vi "FillSurfaceRect.vi"(7 "Entire Surface (F)":bool, 8 "No Error":errorcluster, 9 "color":u32, 10 "rect":T1, 11 "dst [SDL_Surface *]":i64) -> (0 "error out":errorcluster)   [LabVIEW 2024, in "SDL3.lvlib" / "Surface.lvlib"]
doc: "<B>Summary</B>\nPerform a fast fill of a rectangle with a specific color.\n\n<B>Remarks</B>\ncolor should be a pixel of the format used by the surface, and can be generated by SDL_MapRGB() or SDL_MapRGBA(). If the color value contains an alpha component then the destination is simply filled with that alpha information, no blending takes place.\n\nIf there is a clip rectangle set on the destination (set via SDL_SetSurfaceClipRect()), then this function will fill based on the intersection of the clip rectangle and rect."
uses:
  Surface.lvlib
  Rect/Rect--cluster.ctl
  Error/Error.lvlib
  Lib/SDL3-32.dll
  Rect/Rect.lvlib
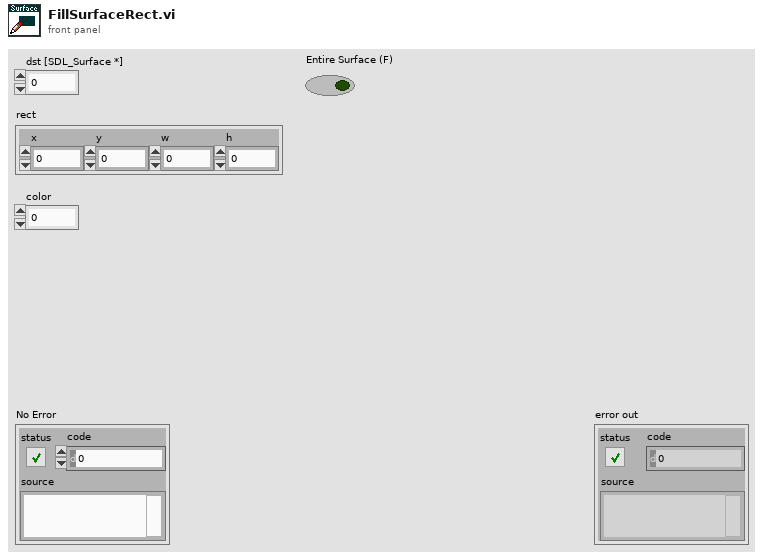
[diagram p1: front panel]
types:
  T1 = typedef "SDL3.lvlib/Rect.lvlib/Rect--cluster.ctl" = cluster{"x":i32, "y":i32, "w":i32, "h":i32}
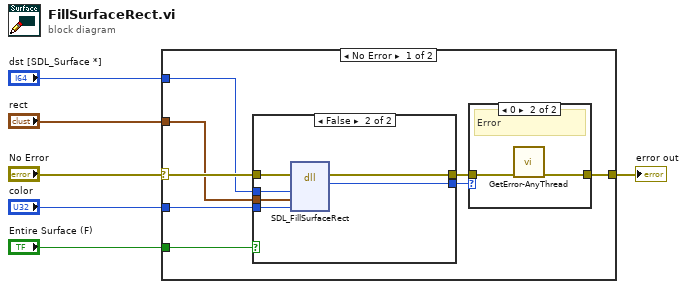
[diagram p0: block diagram]
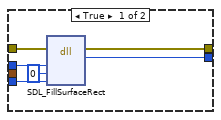
[diagram p2: hidden frame]
diagram:
  n1 = case shown="No Error" "No Error" {
    selector: "No Error" -> [w14 w30]
    tunnel: [w12 w30] -> w5
    tunnel: "dst [SDL_Surface *]" -> [w10 _]
    tunnel: "rect" -> [w9 _]
    tunnel: "color" -> [w8 _]
    tunnel: "Entire Surface (F)" -> [w7 _]
    frame No Error {
      n2 = case shown="False" w7 {
        tunnel: w14 -> [w20 w26]
        tunnel: [w19 w25] -> w13
        tunnel: [w18 w24] -> w11
        tunnel: w10 -> [w17 w23]
        tunnel: w9 -> [_ w22]
        tunnel: w8 -> [w16 w21]
        frame True {
          n3 = dll-call lib="C:/Users/Thomas/Documents/Projects/LV-SDL3/Lib/SDL3-*.*" fn="SDL_FillSurfaceRect"(error in=w20, "dst"=w17, "rect"=i64 0, "color"=w16) -> (error out=w19:errorcluster, "return type"=w18:i32)  [unwired: 5 in, 1 out]
        }
        frame False {
          n4 = dll-call lib="C:/Users/Thomas/Documents/Projects/LV-SDL3/Lib/SDL3-*.*" fn="SDL_FillSurfaceRect"(error in=w26, "dst"=w23, "rect"=w22, "color"=w21) -> (error out=w25:errorcluster, "return type"=w24:i32)  [unwired: 5 in, 1 out]
        }
      }
      n5 = case shown="0" w11 {
        tunnel: w13 -> [w27 w29]
        tunnel: [w27 w28] -> w12
        frame Default {
          # "Ok"
        }
        frame 0 {
          # "Error"
          n6 = call "GetError-AnyThread.vi"("No Error"=w29) -> ("error out"=w28:errorcluster)  [unwired: 10 in]
        }
      }
    }
    frame Error {
    }
  }
  "error out" <- w5
